vi "RGA_scan_new_version_2.vi"(4 "Run Scan?":bool, 7 "Input Parameters":string, 8 "Current Iteration":i32, 9 "Previous Loop Avg.":dbl, 10 "Previous Loop Sum":dbl format="%#_13g", 11 "Current Pressure Reading":dbl) -> (0 "Average Press.  < 2.2E-4 Torr?":bool, 1 "Running Average":dbl, 2 "Running Sum":dbl)   [LabVIEW 2018]
panel:
  out "standard output":string
  out "standard error":string
  out "Average Press [Torr]":dbl
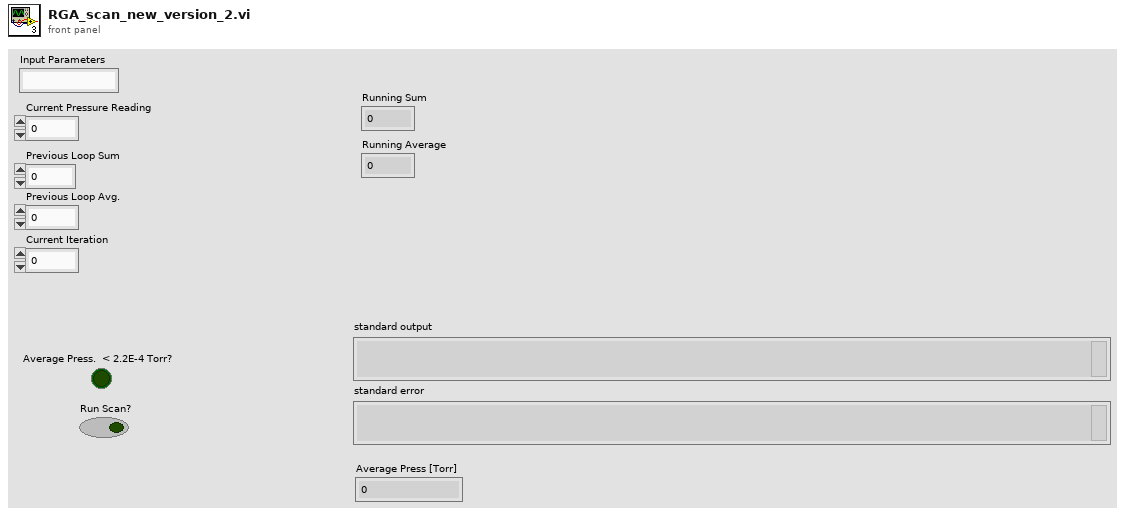
[diagram p1: front panel]
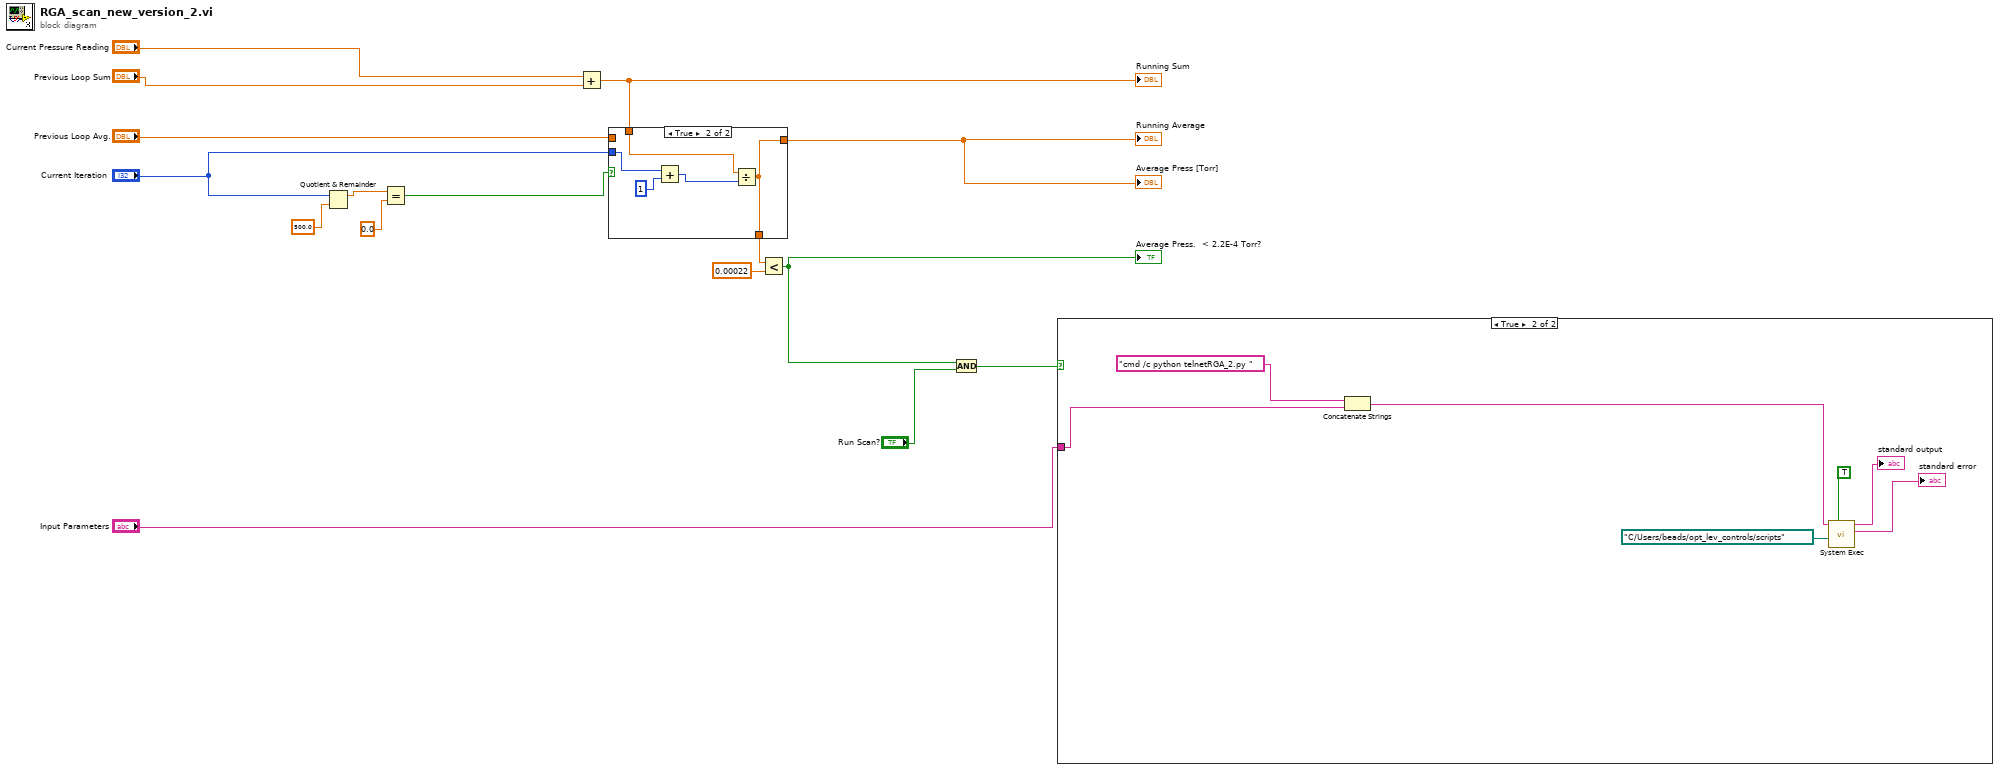
[diagram p0: block diagram]
diagram:
  n1 = Quotient & Remainder(x="Current Iteration", y=500.0) -> (x-y*floor(x/y)=w13:dbl)  [unwired: 1 out]
  n2 = Equal?(x=w13, y=0.0) -> (x = y?=w11:bool)
  n3 = Add(x="Current Pressure Reading", y="Previous Loop Sum") -> (x+y=w15:dbl)
  "Running Sum" <- w15
  n4 = case shown="True" w11 {
    tunnel: "Current Iteration" -> [_ w22]
    tunnel: w15 -> [_ w20]
    tunnel: [w17 w18] -> w6
    tunnel: "Previous Loop Avg." -> [w17 _]
    tunnel: [w17 w18] -> w10
    frame False {
    }
    frame True {
      n5 = Add(x=w22, y=1) -> (x+y=w19:i32)
      n6 = Divide(x=w20, y=w19) -> (x/y=w18:dbl)
    }
  }
  "Average Press [Torr]" <- w6
  "Running Average" <- w6
  n7 = Less?(x=w10, y=0.00022) -> (x < y?=w2:bool)
  "Average Press.  < 2.2E-4 Torr?" <- w2
  n8 = And(x=w2, y="Run Scan?") -> (x .and. y?=w7:bool)
  n9 = case shown="True" w7 {
    tunnel: "Input Parameters" -> [_ w24]
    frame False {
    }
    frame True {
      n10 = Concatenate Strings("cmd /c python telnetRGA_2.py " ("command line"), w24) -> (w23:string)
      n11 = call <vilib>:"System Exec.vi"("wait until completion? (T)"=TRUE, "working directory"=path "C:/Users/beads/opt_lev_controls/scripts", "command line"=w23) -> ("standard error"=→"standard error":string, "standard output"=→"standard output":string)  [unwired: 5 in, 2 out]
    }
  }
